vi "Init Controller.vi"(8 "error in (no error)":errorcluster, 10 "CAN Offset":u32 format="%x", 11 "interface object in":refnum<k20>) -> (0 "error out":errorcluster, 3 "interface object out":refnum<k20>)   [LabVIEW 2014]
uses:
  <vilib>/RioEmbeddedCAN/RioEmbeddedCAN.llb/CANFrameControl.ctl
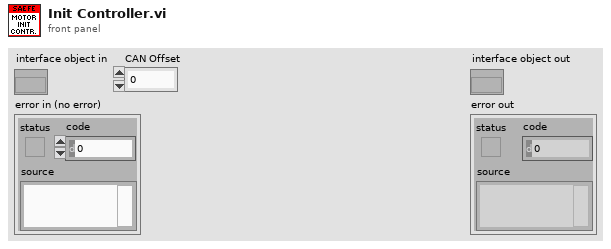
[diagram p1: front panel]
types:
  T1 = typedef "CANFrameControl.ctl" = cluster{"identifier":u32, "extended?":bool, "type":u8, "payload":u8[]}
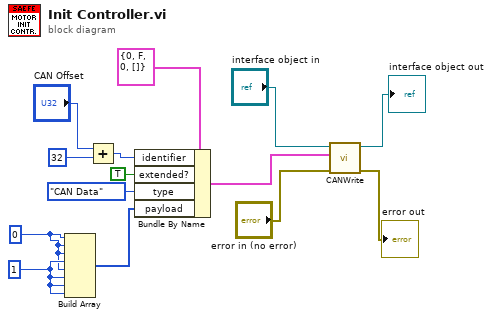
[diagram p0: block diagram]
diagram:
  w4 = u8 1 ("element")
  w3 = u8 0
  n1 = Build Array(w3, w3, w3, w4, w3, w4, w4, w4) -> (w8:u8[])
  n2 = Add(x="CAN Offset", y=u32 32 ("identifier")) -> (x+y=w6:u32)
  n3 = Bundle By Name(cluster=T1 {"identifier"=0, "extended?"=FALSE, "type"=0, "payload"=[]} ("CAN frame"), "identifier"=w6, "extended?"=TRUE, "type"=enum8{"CAN Data", "CAN Remote"}."CAN Data", "payload"=w8) -> (w11:T1)
  n4 = call <vilib>:"CANWrite.vi"("error in (no error)"="error in (no error)", "CAN frame"=w11, "interface object in"="interface object in") -> ("error out"=→"error out":errorcluster, "interface object out"=→"interface object out":refnum<k20>)  [unwired: 7 in]
